vi "Cal1-GetPath.vi"(11 "Calib file":path) -> (1 "String output":string, 2 "exists?":bool, 3 "Path output":path)   [LabVIEW 2016]
uses:
  Anemometry Sub Vis/Globals/Meas_global.vi
  Anemometry Sub Vis/Globals/Calib_global.vi
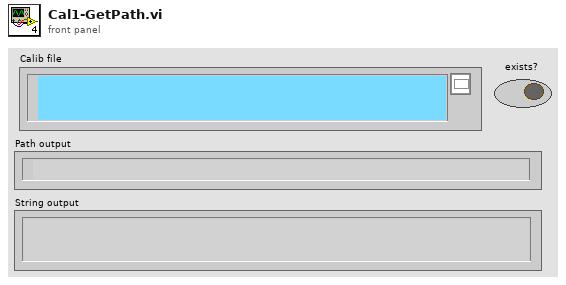
[diagram p1: front panel]
types:
  T1 = enum32{"existing file", "new file", "new or existing file", "existing dir", "new dir", "new or existing dir", "existing file (use LLBs)", "new file (use LLBs)", "new or existing file (use LLBs)", "new or existing file or directory (use LLBs)"}
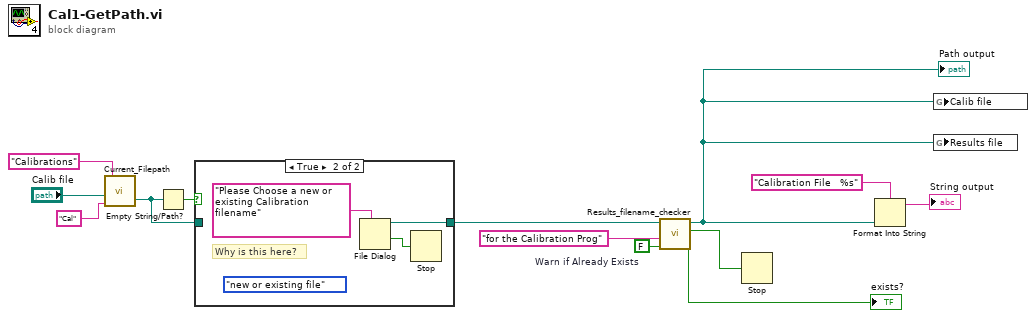
[diagram p0: block diagram]
diagram:
  w2 = FALSE  # Warn if Already Exists
  n1 = call "Current_Filepath.vi"("Short_Name"="Cal" ("Data Type"), "Filename in"="Calib file", "Data Type"="Calibrations") -> ("Filename Out"=w11:path)  [unwired: 1 in, 1 out]
  n2 = Empty String/Path?(string/path=w11) -> (empty?=w6:bool)
  n3 = case shown="True" w6 {
    tunnel: w11 -> [w14 _]
    tunnel: [w14 w16] -> w4
    frame False {
    }
    frame True {
      (unwired) T1."new or existing file" ("select mode (2)")
      # "Why is this here?"
      n4 = File Dialog(7:"Please Choose a new or existing Calibration filename" ("Promp if not found")) -> (1:w15:bool, 3:w16:path)  [unwired: 1 in, 7 out]
      n5 = Stop(stop? (T)=w15) -> ()
    }
  }
  n6 = call "Results_filename_checker.vi"("Warn if Already Exists"=w2, "Comment"="for the Calibration Prog", "Results file"=w4) -> ("exists?"=→"exists?":bool, "cancelled"=w5:bool, "Results file output"=w8:path)  [unwired: 2 in, 1 out]
  "Path output" <- w8
  n7 = Stop(stop? (T)=w5) -> ()
  n8 = Format Into String(format string="Calibration File   %s", w8) -> (resulting string=→"String output":string)  [unwired: 2 in, 1 out]
  n9 = global write "Calib_global.vi" "Calib file"(w8) -> ()
  n10 = global write "Meas_global.vi" "Results file"(w8) -> ()
